vi "SVT Telecommunications Weighting Filter (Fixed Rates).vi"   [LabVIEW 2017, in "SoundVib_TeleWeighting.lvlib"]
doc: "Applies the selected telecommunications weighting filter to a single waveform or multiple waveforms. This VI complies with ITU-T O.41 and Bell System Technical Reference 41009 standards. Each instance of this VI maintains its own state; use the N Waveforms instance of this VI to process an array of channels. This VI operates on time-continuous data; it resets on a discontinuity. Wire data to the<B> scaled signal [EU]</B> input to determine the polymorphic instance to use or manually select the instance."
uses:
  <vilib>/addons/Sound and Vibration/svt_Weighting/SoundVib_TeleWeighting.lvlib
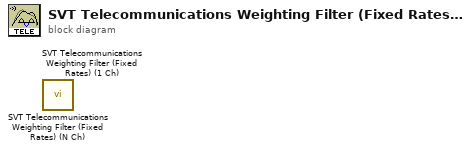
[diagram p0: block diagram]
diagram:
  n1 = call <vilib>:"SVT Telecommunications Weighting Filter (Fixed Rates) (N Ch).vi"() -> ()  [unwired: 9 in, 2 out]
  n2 = call <vilib>:"SVT Telecommunications Weighting Filter (Fixed Rates) (1 Ch).vi"() -> ()  [unwired: 9 in, 2 out]
